vi "Open Ref from Path.vi"(8 "error in (no error)":errorcluster, 11 "VI Reference Control in":refnum<class "VI Reference Control.lvclass">) -> (0 "error out":errorcluster, 3 "VI Reference Control out":refnum<class "VI Reference Control.lvclass">)   [LabVIEW 2016, in "VI Reference Control.lvclass"]
uses:
  VI Reference Control.lvclass
  C:/Users/tblair/Documents/Git Projects/Drag and Drop VI Tool/Reference Control/Reference Control.lvclass
  Reference Control/Reference Control.lvclass/Reference Control.ctl
  VI Reference Control.lvclass/VI Reference Control.ctl
  Reference Control/Read Path Control Ref.vi
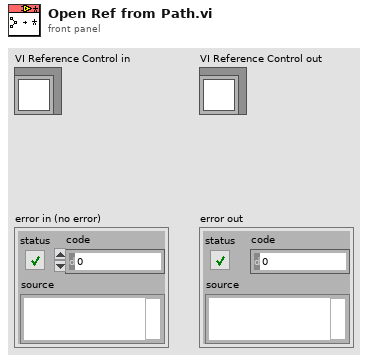
[diagram p1: front panel]
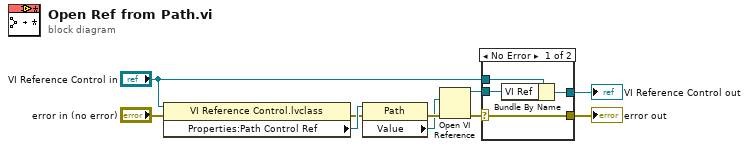
[diagram p0: block diagram]
diagram:
  n1 = property class="VI Reference Control.lvclass"(reference="VI Reference Control in", error in="error in (no error)") -> (error out=w1:errorcluster, "Properties:Path Control Ref"=w3:refnum<vi>)  [unwired: 1 out]
  n2 = property on="Property Node" class="Path"(reference=w3, error in=w1) -> (error out=w8:errorcluster, "Value"=w7:path)  [unwired: 1 out]
  n3 = Open VI Reference(vi path=w7, error in (no error)=w8) -> (vi reference=w9:refnum<vi>, error out=w6:errorcluster)  [unwired: 4 in]
  n4 = case shown="No Error" w6 {
    selector: w6 -> [w11 w16]
    tunnel: [w14 w15] -> w10
    tunnel: w9 -> [w13 _]
    tunnel: "VI Reference Control in" -> [w12 w15]
    tunnel: [w11 w16] -> w5
    frame No Error {
      n5 = Bundle By Name(cluster=w12, "VI Ref"=w13) -> (w14:refnum<class "VI Reference Control.lvclass">)
    }
    frame Error {
    }
  }
  "error out" <- w5
  "VI Reference Control out" <- w10
